vi "Do Commands.vi"(5 "VolatusAPI":refnum<class "VolatusAPI.lvclass">, 6 "State Loop Data in":T1, 11 "State in":refnum<class "State.lvclass">) -> (3 "State out":refnum<class "State.lvclass">, 4 "State Loop Data":T1)   [LabVIEW 2023, in "VolatusSeq.lvlib" / "State.lvclass"]
uses:
  State.lvclass
  State Loop Data.ctl
  Iteration Actions/Iteration Actions.lvclass
  Variables/Variables.lvclass
  Command.ctl
  Volatus/MessageQ/MessageQ.lvclass
  Format String/Format String.lvclass
  VolatusSeqConfig/Command Type.ctl
  messages/CmdDigital/Data.ctl
  messages/CmdAnalog/Data.ctl
  Send Type.ctl
  lv-vecto/Vecto/Channel DBL/Channel DBL.lvclass
  Transition/Transition.lvclass
  Sequence Time.ctl
  VolatusSeqConfig/Debug Flags.ctl
  Volatus/VolatusAPI/VolatusAPI.lvclass
  Iteration Actions/Iteration Actions.lvclass/Iteration Actions.ctl
  messages/CmdDigitalMultiple/Class/Msg.lvclass/Msg.ctl
  Volatus/VolatusAPI/VolatusAPI.lvclass/VolatusAPI.ctl
  messages/CmdAnalogMultiple/Class/Msg.lvclass/Msg.ctl
  Volatus/MessageQ/MessageQ.lvclass/MessageQ.ctl
  messages/CmdDigitalMultiple/Class/Msg.lvclass
  C:/dev/volatus/mts-volatus-super/libs/lv-protoc/LV-Proto/Message/Message.lvclass
  messages/CmdAnalogMultiple/Class/Msg.lvclass
  lv-vecto/Vecto/TCPMessageService/Send Message.vi
  <vilib>/Utility/error.llb/Error Cluster From Error Code.vi
  lv-protoc/LV-Proto/Message/Message.lvclass
  VolatusSeq.lvlib
  VolatusSeqConfig/VolatusSeqConfig.lvlib
  messages/CmdDigital/CmdDigital.lvlib
  messages/CmdAnalog/CmdAnalog.lvlib
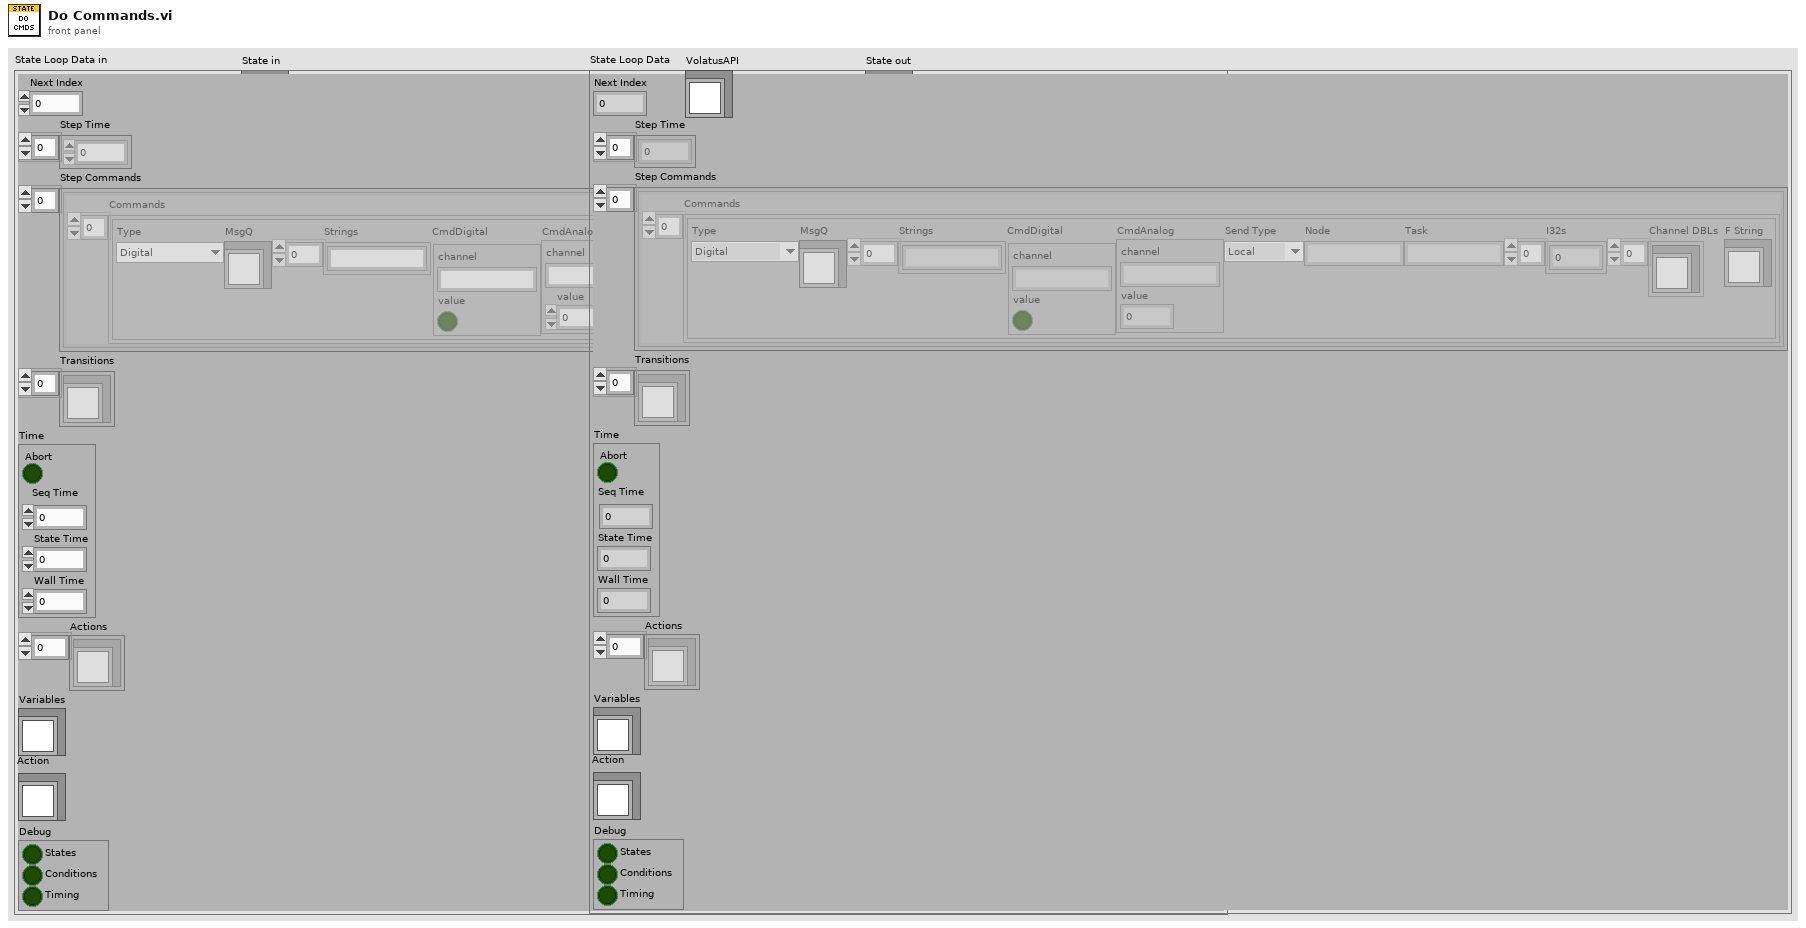
[diagram p1: front panel]
types:
  T1 = typedef "VolatusSeq.lvlib/State.lvclass/State Loop Data.ctl" = cluster{"Next Index":i32, "Step Time":dbl[], "Step Commands":cluster{"Commands":T2[]}[], "Transitions":refnum<class "Transition.lvclass">[], "Time":T7, "Actions":refnum<class "Iteration Actions.lvclass">[], "Variables":refnum<class "Variables.lvclass">, "Action":refnum<class "Iteration Actions.lvclass">, "Debug":T8}
  T2 = typedef "VolatusSeq.lvlib/Command.ctl" = cluster{"Type":T3, "MsgQ":refnum<class "MessageQ.lvclass">, "Strings":string[], "CmdDigital":T4, "CmdAnalog":T5, "Send Type":T6, "Node":string, "Task":string, "I32s":i32[], "Channel DBLs":refnum<class "Channel DBL.lvclass">[], "F String":refnum<class "Format String.lvclass">}
  T3 = typedef "VolatusSeqConfig.lvlib/Command Type.ctl" = enum16{"Digital", "Numeric", "Transition", "Stop", "StartLog", "StopLog", "Start", "Event", "Error", "HTTP", "ResetVar", "IncVar", "DecVar", "SaveVar", "LoadVar", "AddVar", "SubVar", "SetVar", "AddToVar"}
  T4 = typedef "CmdDigital.lvlib/Data.ctl" = cluster{"channel":string, "value":bool}
  T5 = typedef "CmdAnalog.lvlib/Data.ctl" = cluster{"channel":string, "value":dbl}
  T6 = typedef "VolatusSeq.lvlib/Send Type.ctl" = enum16{"Local", "Remote"}
  T7 = typedef "VolatusSeq.lvlib/Sequence Time.ctl" = cluster{"Abort":bool, "Seq Time":dbl, "State Time":dbl, "Wall Time":dbl}
  T8 = typedef "VolatusSeqConfig.lvlib/Debug Flags.ctl" = cluster{"States":bool, "Conditions":bool, "Timing":bool}
  T9 = typedef "CmdAnalogMultiple.lvlib/Data.ctl" = cluster{"values":T5[]}
  T10 = typedef "CmdDigitalMultiple.lvlib/Data.ctl" = cluster{"values":T4[]}
  T11 = typedef "VolatusSeq.lvlib/Remote Analog.ctl" = cluster{"Node":string, "Cmd":T9}
  T12 = typedef "VolatusSeq.lvlib/Remote Digital.ctl" = cluster{"Node":string, "Cmd":T10}
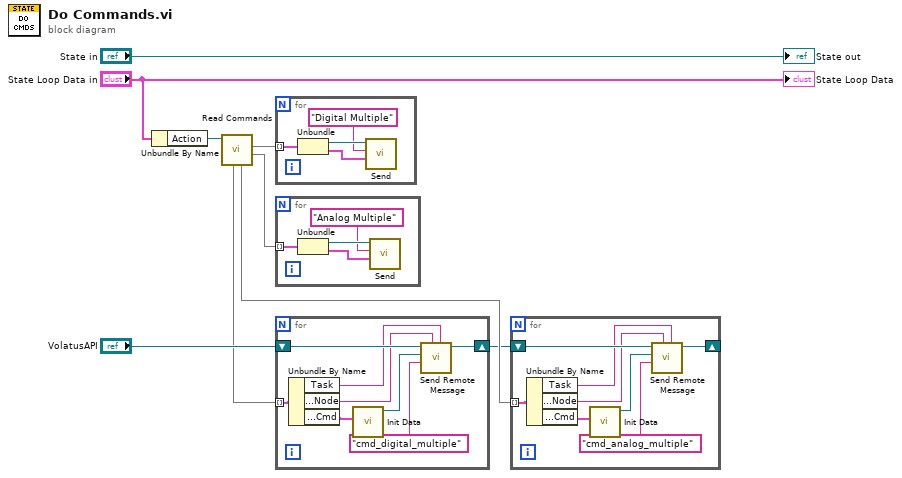
[diagram p0: block diagram]
diagram:
  n1 = Unbundle By Name("State Loop Data in") -> ("Action"=w1:refnum<class "Iteration Actions.lvclass">)
  n2 = call "Read Commands.vi"("Iteration Actions in"=w1) -> ("Analog Commands"=w5:map{refnum<class "MessageQ.lvclass">, T9}, "Digital Commands"=w6:map{refnum<class "MessageQ.lvclass">, T10}, "Remote Analog"=w3:map{string, T11}, "Remote Digital"=w4:map{string, T12})  [unwired: 5 in, 2 out]
  n3 = for {
    tunnel: w6 -> [w13] mode=indexing
    n4 = Unbundle(w13) -> ("MsgQ"=w12:refnum<class "MessageQ.lvclass">, "CmdDigitalMultiple"=w10:T10)
    n5 = call "Send.vi"("Data"=w10, "ID"="Digital Multiple", "MessageQ in"=w12) -> ()  [unwired: 7 in, 2 out]
  }
  n6 = for {
    tunnel: w5 -> [w17] mode=indexing
    n7 = Unbundle(w17) -> ("MsgQ"=w16:refnum<class "MessageQ.lvclass">, "CmdAnalogMultiple"=w14:T9)
    n8 = call "Send.vi"("Data"=w14, "ID"="Analog Multiple", "MessageQ in"=w16) -> ()  [unwired: 7 in, 2 out]
  }
  n9 = for {
    shift-right: [w21] -> w2
    shift-left: "VolatusAPI" -> [w24]
    tunnel: w4 -> [w25] mode=indexing
    n10 = Unbundle By Name(w25) -> ("Task"=w23:string, "Command.Node"=w22:string, "Command.Cmd"=w19:T10)
    n11 = call "Init Data.vi"("Data"=w19) -> ("Msg out"=w18:refnum<class "Msg.lvclass">)  [unwired: 10 in]
    n12 = call "Send Remote Message.vi"("Target Task (None)"=w23, "Target Name"=w22, "Message Type"="cmd_digital_multiple", "Message"=w18, "VolatusAPI in"=w24) -> ("VolatusAPI out"=w21:refnum<class "VolatusAPI.lvclass">)  [unwired: 5 in, 1 out]
  }
  n13 = for {
    shift-right: [w29] -> _
    shift-left: w2 -> [w32]
    tunnel: w3 -> [w33] mode=indexing
    n14 = Unbundle By Name(w33) -> ("Task"=w31:string, "Command.Node"=w30:string, "Command.Cmd"=w27:T9)
    n15 = call "Init Data.vi"("Data"=w27) -> ("Msg out"=w26:refnum<class "Msg.lvclass">)  [unwired: 10 in]
    n16 = call "Send Remote Message.vi"("Target Task (None)"=w31, "Target Name"=w30, "Message Type"="cmd_analog_multiple", "Message"=w26, "VolatusAPI in"=w32) -> ("VolatusAPI out"=w29:refnum<class "VolatusAPI.lvclass">)  [unwired: 5 in, 1 out]
  }
  "State out" <- "State in"
  "State Loop Data" <- "State Loop Data in"
